vi "NodeSkip.vi"(10 "Node":dbl[](array[numeric]), 11 "Signal?":bool=TRUE) -> (3 "Skip":i32)   [LabVIEW 2020]
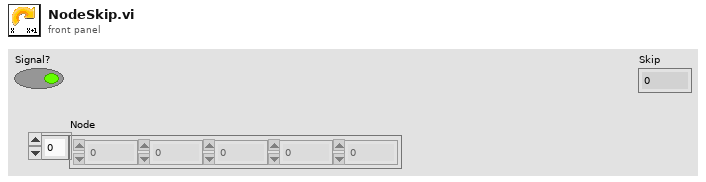
[diagram p1: front panel]
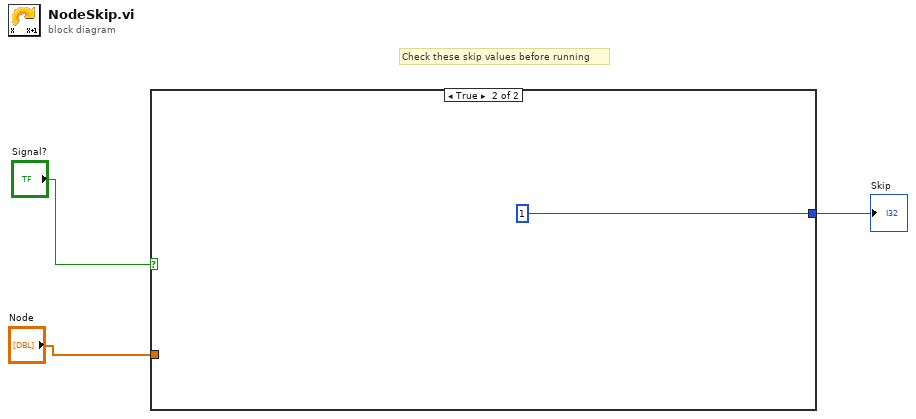
[diagram p0: block diagram]
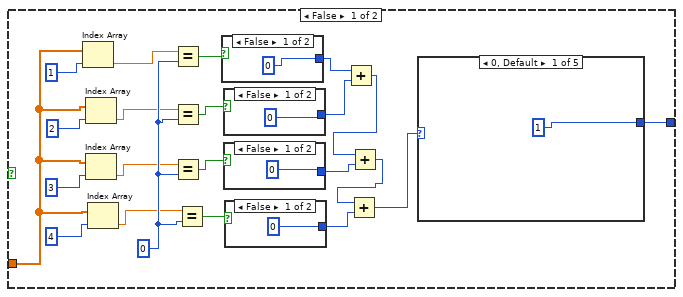
[diagram p2: hidden frame]
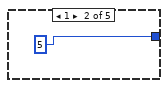
[diagram p3: hidden frame]
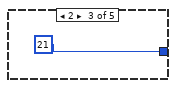
[diagram p4: hidden frame]
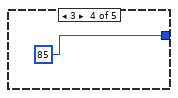
[diagram p5: hidden frame]
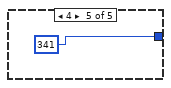
[diagram p6: hidden frame]
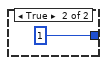
[diagram p7: hidden frame]
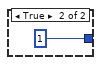
[diagram p8: hidden frame]
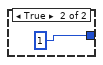
[diagram p9: hidden frame]
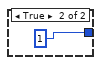
[diagram p10: hidden frame]
diagram:
  # "Check these skip values before running"
  n1 = case shown="True" "Signal?" {
    tunnel: "Node" -> [w24 _]
    tunnel: [w4 1] -> w1
    frame False {
      w20 = 0
      n2 = Index Array(array=w24, index=1) -> (element=w16:dbl)
      n3 = Index Array(array=w24, index=2) -> (element=w17:dbl)
      n4 = Index Array(array=w24, index=3) -> (element=w18:dbl)
      n5 = Index Array(array=w24, index=4) -> (element=w19:dbl)
      n6 = Equal?(x=w16, y=w20) -> (x = y?=w15:bool)
      n7 = Equal?(x=w17, y=w20) -> (x = y?=w14:bool)
      n8 = Equal?(x=w18, y=w20) -> (x = y?=w13:bool)
      n9 = Equal?(x=w19, y=w20) -> (x = y?=w12:bool)
      n10 = case shown="False" w15 {
        tunnel: [0 1] -> w11
        frame False {
        }
        frame True {
        }
      }
      n11 = case shown="False" w14 {
        tunnel: [0 1] -> w10
        frame False {
        }
        frame True {
        }
      }
      n12 = case shown="False" w13 {
        tunnel: [0 1] -> w8
        frame False {
        }
        frame True {
        }
      }
      n13 = case shown="False" w12 {
        tunnel: [0 1] -> w6
        frame False {
        }
        frame True {
        }
      }
      n14 = Add(x=w11, y=w10) -> (x+y=w9:i32)
      n15 = Add(x=w9, y=w8) -> (x+y=w7:i32)
      n16 = Add(x=w7, y=w6) -> (x+y=w5:i32)
      n17 = case shown="0, Default" w5 {
        tunnel: [1 5 21 85 341] -> w4
        frame 0, Default {
        }
        frame 1 {
        }
        frame 2 {
        }
        frame 3 {
        }
        frame 4 {
        }
      }
    }
    frame True {
    }
  }
  "Skip" <- w1
